vi "AutoUpdateState.vi"(3 "Ïµ½y î‘B":refnum<vi>, 4 "ê ÁÐ”µ“þ":cluster{"State":T1, "Data":string}={"State"=enum."Quit", "Data"=""}) -> (1 "ê ÁÐ”µ“þ":cluster{"State":T1, "Data":string}={"State"=enum."Quit", "Data"=""})   [LabVIEW 2012]
uses:
  SystemState.ctl
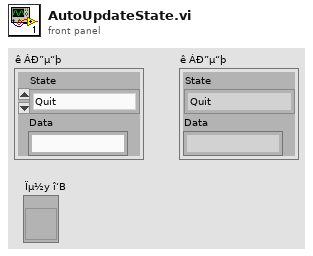
[diagram p1: front panel]
types:
  T1 = typedef "SystemState.ctl" = enum16{"Pause", "Quit", "Error", "Stopping", "Starting", "Init", "Scan", "Menu", "ReadConf", "Idle"}
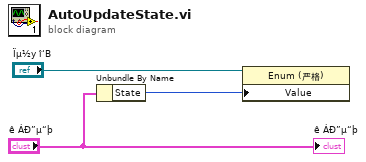
[diagram p0: block diagram]
diagram:
  n1 = Unbundle By Name("ê ÁÐ”µ“þ") -> ("State"=w1:T1)
  n2 = property class="Enum (严格)"(reference="Ïµ½y î‘B", "Value"=w1) -> ()  [unwired: 1 in, 2 out]
  "ê ÁÐ”µ“þ" <- "ê ÁÐ”µ“þ"
